vi "make single scan multivariable array string.vi"(6 "precision other (12)":i16, 9 "P(x)":dbl[][](array[numeric])=[[-1.74, 0.00227273], [1.07, -0.00113636]] caption="P(x) ascending order of power." min=0.0 max=127.0 format="%#.6f", 10 "Cluster":T2 {"Scan parameters"."Scan Start" format="%#.9p"; "Scan parameters"."Scan End" format="%#.9p"; "Scan parameters"."Scan Step Size" format="%#.9p"}, 11 "precision primary":i16) -> (3 "String":string)   [LabVIEW 2013]
uses:
  scan parameters.ctl
  <vilib>/Analysis/1siggen.llb/Ramp Pattern by Delta.vi
  <vilib>/Analysis/polynomials.llb/1D Polynomial Evaluation (DBL).vi
  <vilib>/Analysis/NI_AALBase.lvlib
  <vilib>/Analysis/NI_AALPro.lvlib
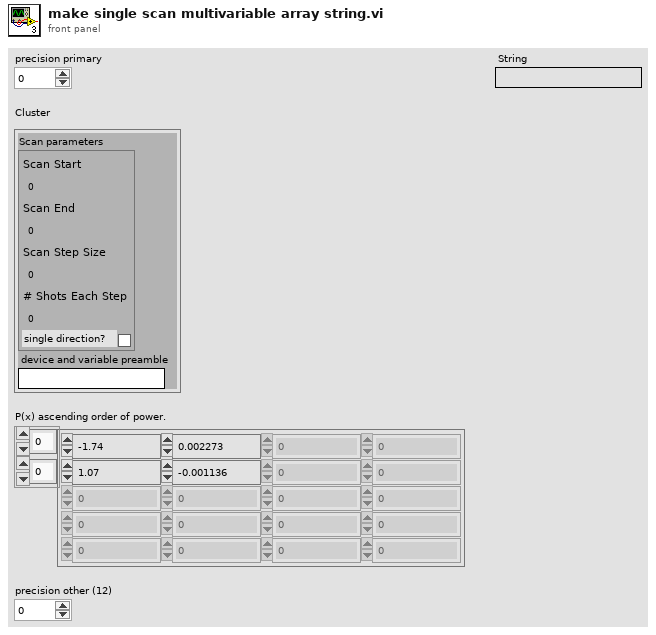
[diagram p1: front panel]
types:
  T1 = typedef "scan parameters.ctl" = cluster{"Scan Start":dbl, "Scan End":dbl, "Scan Step Size":dbl, "# Shots Each Step":u32, "single direction?":bool}
  T2 = cluster{"Scan parameters":T1, "device and variable preamble":string}
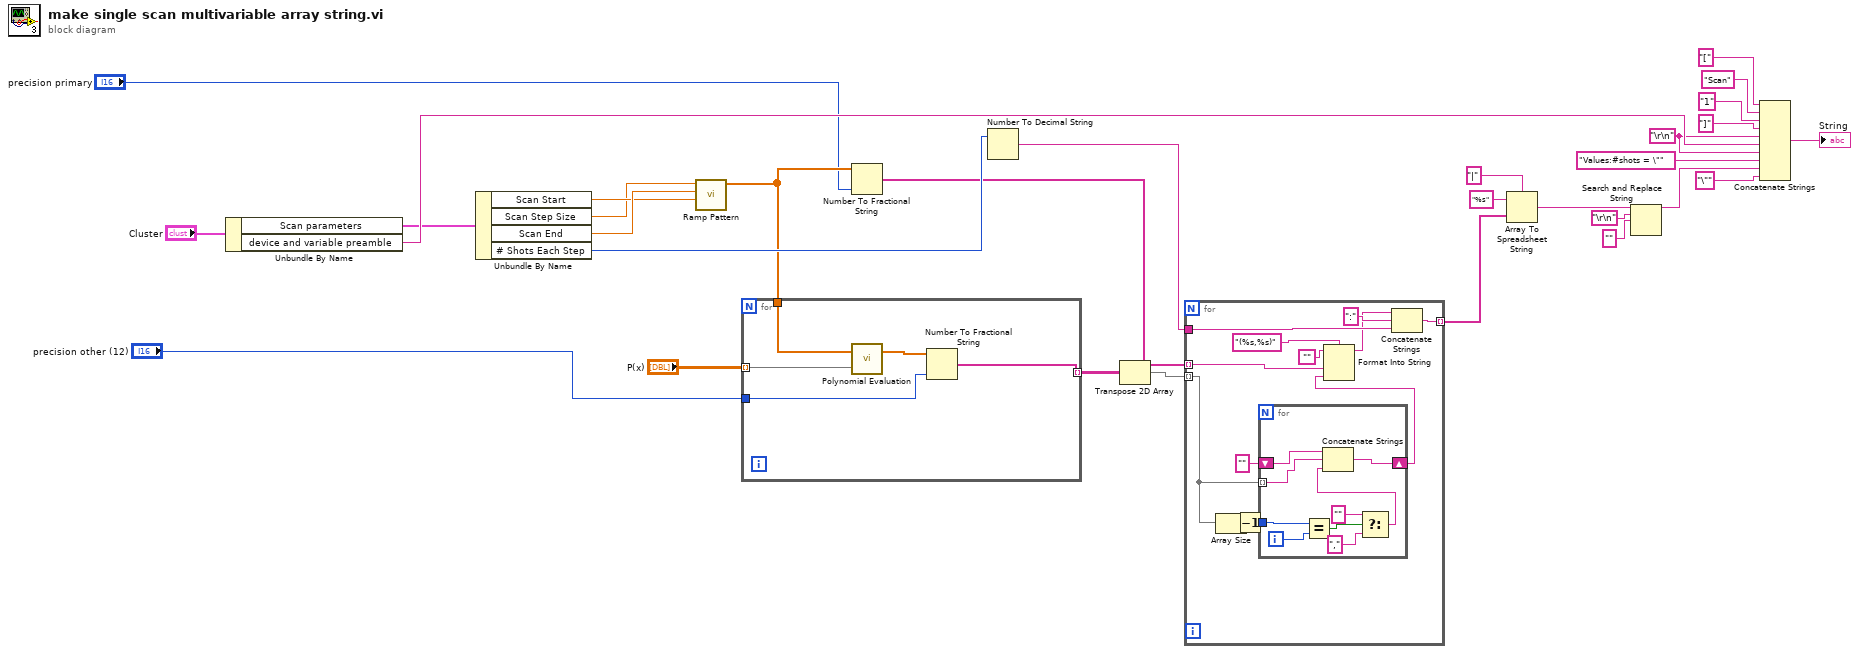
[diagram p0: block diagram]
diagram:
  w2 = "\r\n"
  n1 = Unbundle By Name("Cluster") -> ("Scan parameters"=w21:T1, "device and variable preamble"=w23:string)
  n2 = Unbundle By Name(w21) -> ("Scan Start"=w10:dbl, "Scan Step Size"=w9:dbl, "Scan End"=w11:dbl, "# Shots Each Step"=w26:u32)
  n3 = call-poly <vilib>:"Ramp Pattern.vi"("start"=w10, "end"=w11, "delta"=w9) -> ("Ramp Pattern"=w24:dbl[])  [unwired: 6 in, 2 out]
  n4 = for {
    tunnel: "precision other (12)" -> [w35]
    tunnel: w24 -> [w34]
    tunnel: "P(x)" -> [w33] mode=indexing
    tunnel: [w32] -> w28 mode=indexing
    n5 = call-poly <vilib>:"Polynomial Evaluation.vi"("P(x)"=w33, "A"=w34) -> ("P(A)"=w31:dbl[])  [unwired: 1 out]
    n6 = Number To Fractional String(number=w31, precision (6)=w35) -> (F-format string=w32:string[])  [unwired: 2 in]
  }
  n7 = Number To Fractional String(number=w24, precision (6)="precision primary") -> (F-format string=w17:string[])  [unwired: 2 in]
  n8 = Number To Decimal String(number=w26) -> (decimal integer string=w13:string)  [unwired: 1 in]
  n9 = Transpose 2D Array(2D array=w28) -> (transposed array=w29:string[][])
  n10 = for {
    tunnel: w17 -> [w43] mode=indexing
    tunnel: w13 -> [w46]
    tunnel: [w45] -> w14 mode=indexing
    tunnel: w29 -> [w38] mode=indexing
    n11 = Array Size(array=w38) -> (size(s)=w37:i32)
    n12 = Decrement(x=w37) -> (x-1=w36:i32)
    n13 = for {
      shift-right: [w56] -> w40
      shift-left: "" -> [w55]
      tunnel: w38 -> [w54] mode=indexing
      tunnel: w36 -> [w52]
      i -> [w53]
      n14 = Equal?(x=w52, y=w53) -> (x = y?=w51:bool)
      n15 = Select(t="", s=w51, f="," ("string")) -> (s? t:f=w48:string)
      n16 = Concatenate Strings(w55, w54, w48) -> (w56:string)
    }
    n17 = Format Into String(format string="(%s,%s)", initial string="", w43, w40) -> (resulting string=w42:string)  [unwired: 1 in, 1 out]
    n18 = Concatenate Strings(w42, ":" ("string"), w46) -> (w45:string)
  }
  n19 = Array To Spreadsheet String(delimiter (Tab)="|", array=w14, 3:"%s" ("format string")) -> (spreadsheet string=w18:string)
  n20 = Search and Replace String(input string=w18, search string="\r\n", replace string="" ("replace string (\"\")")) -> (result string=w22:string)  [unwired: 5 in, 3 out]
  n21 = Concatenate Strings("[" ("string"), "Scan", "1" ("scan #"), "]" ("string"), w2, w23, w2, "Values:#shots = \"" ("string"), w22, "\"" ("string")) -> (→"String":string)
